vi "BASE_Login Screen.vi"(8 "Error In":errorcluster, 10 "Password":string, 11 "User Name":string(combo)) -> (0 "error out":errorcluster, 1 "Level":i32, 2 "Login Done":bool, 3 "User Name Out":string(combo))   [LabVIEW 2017]
uses:
  <vilib>/Utility/config.llb/Read Key (String).vi
  <vilib>/Utility/config.llb/Read Key (I32).vi
  <vilib>/Utility/config.llb/NI_LVConfig.lvlib
panel:
  in  "Cancel":bool
  in  "OK Button":bool
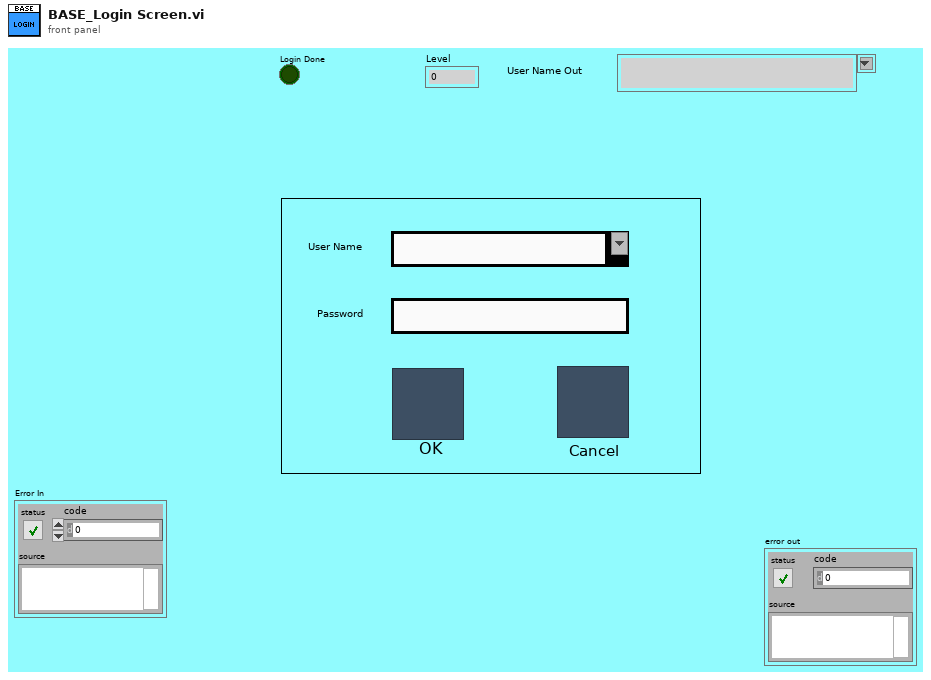
[diagram p1: front panel]
types:
  T1 = enum32{"invalid app kind", "Development System", "Run Time System", "Student Edition", "Embedded LabVIEW", "Evaluation", "Custom"}
  T2 = typedef "NI_LVConfig.lvlib/Config Data RefNum.ctl" = refnum<k1>
  T3 = enum32{"Invalid", "Standard", "Closed", "Hidden", "Minimized", "Maximized"}
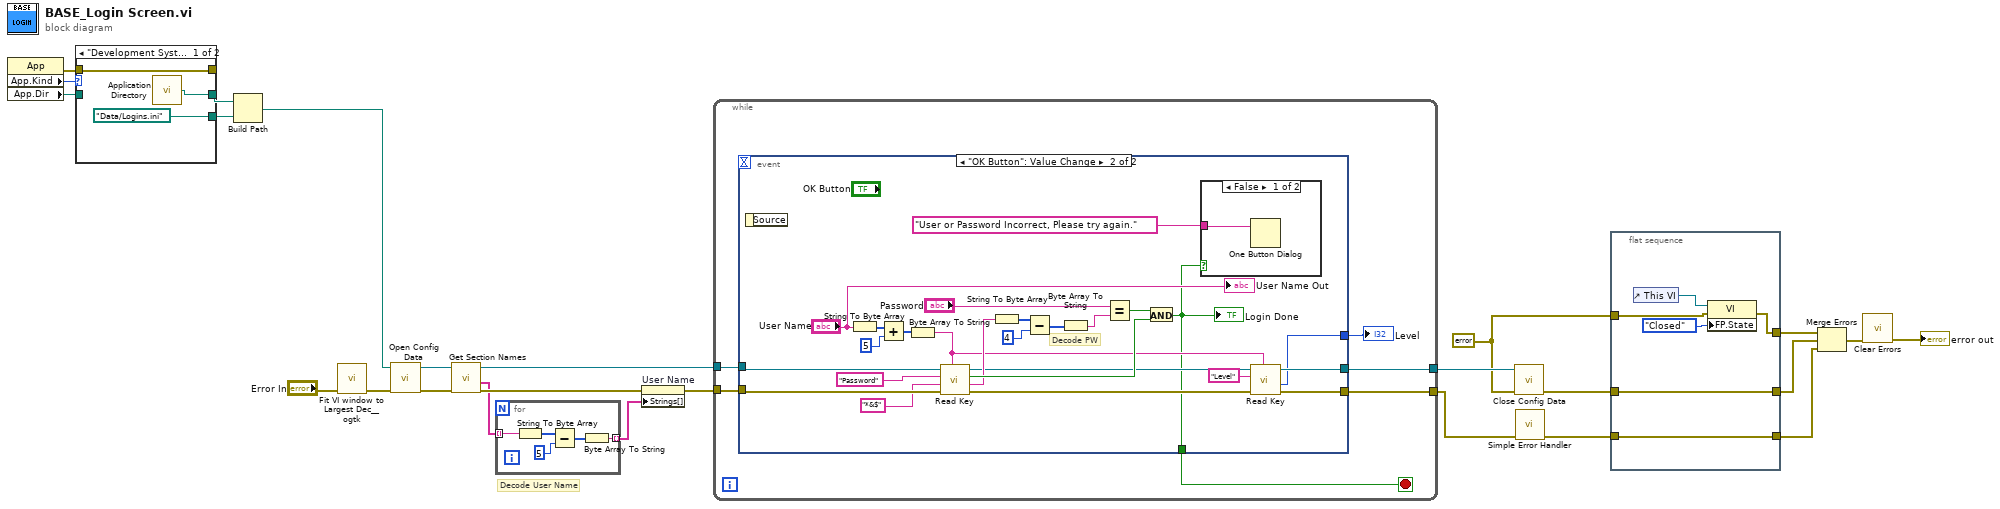
[diagram p0: block diagram]
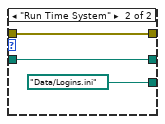
[diagram p2: hidden frame]
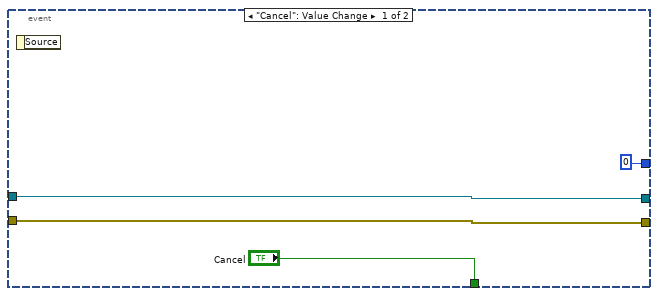
[diagram p3: hidden frame]
diagram:
  w23 = errorcluster {"status"=FALSE, "code"=0, "source"=""} ("error in (no error)")
  # "Decode User Name"
  n1 = property class="App"() -> (error out=w3:errorcluster, "App.Kind"=w6:T1, "App.Dir"=w4:path)  [unwired: 2 in, 1 out]
  n2 = case shown="\"Development System\", Default" w6 {
    tunnel: [w28 w31] -> _
    tunnel: w3 -> [w28 w31]
    tunnel: w4 -> [_ w29]
    tunnel: [path "Data/Logins.ini" path "Data/Logins.ini"] -> w5
    tunnel: [w26 w29] -> w2
    frame "Development System", Default {
      n3 = call <vilib>:"Application Directory.vi"() -> ("Application Directory"=w26:path)
    }
    frame "Run Time System" {
    }
  }
  n4 = Build Path(base path=w2, name or relative path=w5) -> (appended path=w1:path)
  n5 = call <userlib>:"Fit VI window to Largest Dec__ogtk.vi"("error in (no error)"="Error In") -> ("error out"=w7:errorcluster)  [unwired: 5 in, 1 out]
  n6 = call <vilib>:"Open Config Data.vi"("error in (no error)"=w7, "configuration file path"=w1) -> ("error out"=w14:errorcluster, "refnum"=w15:T2)  [unwired: 7 in, 1 out]
  n7 = call <vilib>:"Get Section Names.vi"("error in (no error)"=w14, "refnum"=w15) -> ("error out"=w12:errorcluster, "section names"=w10:string[], "refnum out"=w13:T2)  [unwired: 7 in]
  n8 = for {
    tunnel: w10 -> [w36] mode=indexing
    tunnel: [w32] -> w9 mode=indexing
    n9 = String To Byte Array(string=w36) -> (unsigned byte array=w35:u8[])
    n10 = Subtract(x=w35, y=u8 5) -> (x-y=w33:u8[])
    n11 = Byte Array To String(unsigned byte array=w33) -> (string=w32:string)
  }
  n12 = property on="User Name" class="CmbBox"(error in=w12, "Strings[]"=w9) -> (error out=w11:errorcluster)  [unwired: 1 in, 1 out]
  n13 = while {
    tunnel: [w41] -> w25
    tunnel: w13 -> [w40]
    tunnel: [w39] -> w24
    tunnel: w11 -> [w38]
    stop <- w42 stop-if-true
    n14 = event shown="[1] \"OK Button\": Value Change" {
      selector: _ -> [_ _]
      dyn-events: _ -> [_ _]
      timeout: _ -> [_ _]
      tunnel: ["Cancel" w48] -> w42
      tunnel: [w45 w52] -> w41
      tunnel: w40 -> [w45 w71]
      tunnel: [w44 w51] -> w39
      tunnel: w38 -> [w44 w70]
      tunnel: [0 ("value") w49] -> w37
      event "Cancel": Value Change {
        n15 = event-data() -> ()  [unwired: 1 in, 1 out]
      }
      event "OK Button": Value Change {
        # "Decode PW"
        n16 = event-data() -> ()  [unwired: 1 in, 1 out]
        n17 = String To Byte Array(string="User Name") -> (unsigned byte array=w59:u8[])
        n18 = Add(x=w59, y=u8 5) -> (x+y=w57:u8[])
        n19 = Byte Array To String(unsigned byte array=w57) -> (string=w55:string)
        n20 = call-poly <vilib>:"Read Key.vi"("section"=w55, "error in (no error)"=w70, "default value"="*&$", "key"="Password", "refnum"=w71) -> ("error out"=w54:errorcluster, "value"=w64:string, "found?"=w66:bool, "refnum out"=w53:T2)  [unwired: 3 in]
        n21 = String To Byte Array(string=w64) -> (unsigned byte array=w63:u8[])
        n22 = Subtract(x=w63, y=u8 4) -> (x-y=w61:u8[])
        n23 = Byte Array To String(unsigned byte array=w61) -> (string=w60:string)
        n24 = Equal?(x="Password", y=w60) -> (x = y?=w67:bool)
        n25 = And(x=w67, y=w66) -> (x .and. y?=w48:bool)
        "Login Done" <- w48
        n26 = case shown="False" w48 {
          tunnel: "User or Password Incorrect, Please try again." -> [w72 _]
          frame False {
            n27 = One Button Dialog(message=w72) -> ()  [unwired: 1 in, 1 out]
          }
          frame True {
          }
        }
        n28 = call-poly <vilib>:"Read Key.vi"("section"=w55, "error in (no error)"=w54, "key"="Level", "refnum"=w53) -> ("error out"=w51:errorcluster, "value"=w49:i32, "refnum out"=w52:T2)  [unwired: 4 in, 1 out]
        "User Name Out" <- "User Name"
      }
    }
    "Level" <- w37
  }
  n29 = call <vilib>:"Close Config Data.vi"("error in (no error)"=w23, "refnum"=w25) -> ("error out"=w18:errorcluster)  [unwired: 8 in, 1 out]
  n30 = call <vilib>:"Simple Error Handler.vi"("error in (no error)"=w24) -> ("error out"=w16:errorcluster)  [unwired: 4 in, 4 out]
  n31 = flat-sequence {
    tunnel: w23 -> [w76]
    tunnel: [w75] -> w22
    tunnel: [w74] -> w19
    tunnel: w18 -> [w74]
    tunnel: [w73] -> w17
    tunnel: w16 -> [w73]
    frame #0 {
      n32 = control-ref of="This VI"() -> (w78:refnum<vi>)
      n33 = property class="VI"(reference=w78, error in=w76, "FP.State"=T3."Closed" ("Front Panel Window:State")) -> (error out=w75:errorcluster)  [unwired: 1 out]
    }
  }
  n34 = Merge Errors(w22, w19, w17) -> (w21:errorcluster)
  n35 = call <vilib>:"Clear Errors.vi"("error in (no error)"=w21) -> ("error out"=→"error out":errorcluster)  [unwired: 5 in, 1 out]
